vi "GetAmplitudeScale.vi"(8 "error in (no error)":errorcluster, 11 "metric":T2) -> (0 "error out":errorcluster, 3 "amplitude scale":T1)   [LabVIEW 2017, in "AnalysisHelper.lvlib"]
uses:
  <vilib>/addons/InsightCM/Utilities/Analysis/Shared/AnalysisHelper.lvlib
  <vilib>/addons/InsightCM/MessageBus/Base/controls/Metric.ctl
  <vilib>/addons/InsightCM/MessageBus/Base/controls/KeyValuePair.ctl
  <vilib>/addons/InsightCM/Utilities/Analysis/Shared/controls/AmplitudeScale.ctl
  <vilib>/addons/InsightCM/Utilities/PropertyHelpers/PropertyHelpers.lvlib
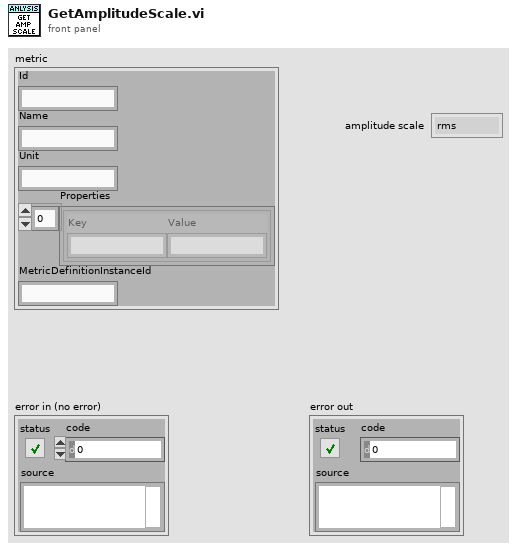
[diagram p1: front panel]
types:
  T1 = typedef "AnalysisHelper.lvlib/AmplitudeScale.ctl" = enum16{"rms", "peak", "pk-pk"}
  T2 = typedef "Metric.ctl" = cluster{"Id":string, "Name":string, "Unit":string, "Properties":T3[], "MetricDefinitionInstanceId":string}
  T3 = typedef "KeyValuePair.ctl" = cluster{"Key":string, "Value":string}
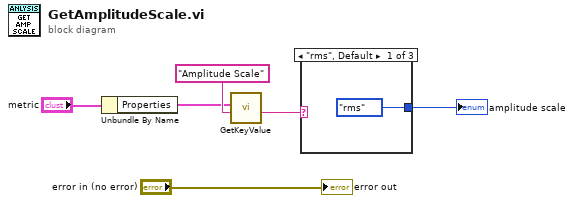
[diagram p0: block diagram]
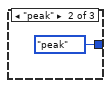
[diagram p2: hidden frame]
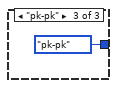
[diagram p3: hidden frame]
diagram:
  n1 = Unbundle By Name("metric") -> ("Properties"=w4:T3[])
  n2 = call <vilib>:"GetKeyValue.vi"("key"="Amplitude Scale", "key value pairs"=w4) -> ("value"=w2:string)  [unwired: 7 in, 2 out]
  n3 = case shown="\"rms\", Default" w2 {
    tunnel: [AmplitudeScale."rms" ("Amplitude Scale") AmplitudeScale."peak" ("Amplitude Scale") AmplitudeScale."pk-pk" ("Amplitude Scale")] -> w1
    frame "rms", Default {
    }
    frame "peak" {
    }
    frame "pk-pk" {
    }
  }
  "amplitude scale" <- w1
  "error out" <- "error in (no error)"
